vi "ConfigBulkSBDDownloadFilenames.vi"(6 "Filenames":string[](array[string]), 9 "Day":string, 10 "Month":string, 11 "Save Path":path) -> (2 "Array":T1(array[cluster]), 3 "dup path":path)   [LabVIEW 2014]
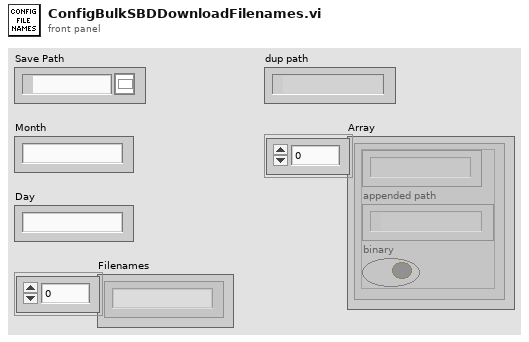
[diagram p1: front panel]
types:
  T1 = cluster{"String":string, "appended path":path, "binary":bool}[]
  T2 = cluster{string, "appended path":path, "binary":bool}
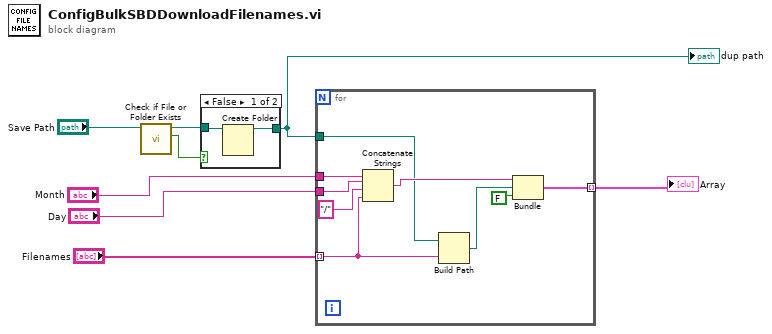
[diagram p0: block diagram]
diagram:
  n1 = call <vilib>:"Check if File or Folder Exists.vi"("path"="Save Path") -> ("file or folder exists?"=w5:bool, "dup path"=w6:path)  [unwired: 8 in, 1 out]
  n2 = case shown="False" w5 {
    tunnel: [w10 w11] -> w8
    tunnel: w6 -> [w9 w11]
    frame False {
      n3 = Create Folder(path (use dialog)=w9) -> (created path=w10:path)  [unwired: 2 in, 2 out]
    }
    frame True {
    }
  }
  "dup path" <- w8
  n4 = for {
    tunnel: "Filenames" -> [w12] mode=indexing
    tunnel: "Day" -> [w19]
    tunnel: w8 -> [w13]
    tunnel: "Month" -> [w18]
    tunnel: [w15] -> w3 mode=indexing
    n5 = Concatenate Strings(w18, w19, "/", w12) -> (w16:string)
    n6 = Build Path(base path=w13, name or relative path=w12) -> (appended path=w14:path)
    n7 = Bundle(w16, "appended path"=w14, "binary"=FALSE) -> (w15:T2)  [unwired: 1 in]
  }
  "Array" <- w3
